vi "BC Wrapper.vi"(0 "File To Program":path, 7 "BootCommander Folder":path, 11 "Error In":errorcluster) -> (4 "StdOut":string, 6 "Std Error":string, 15 "error out":errorcluster)   [LabVIEW 2021]
doc: "It's wrapper for the BootCommander.exe"
uses:
  Controls/Console Manager Functions.ctl
  <vilib>/JKI/JKI DotNet System Exec/dotnet_system_exec/dotnet_system_exec.lvclass
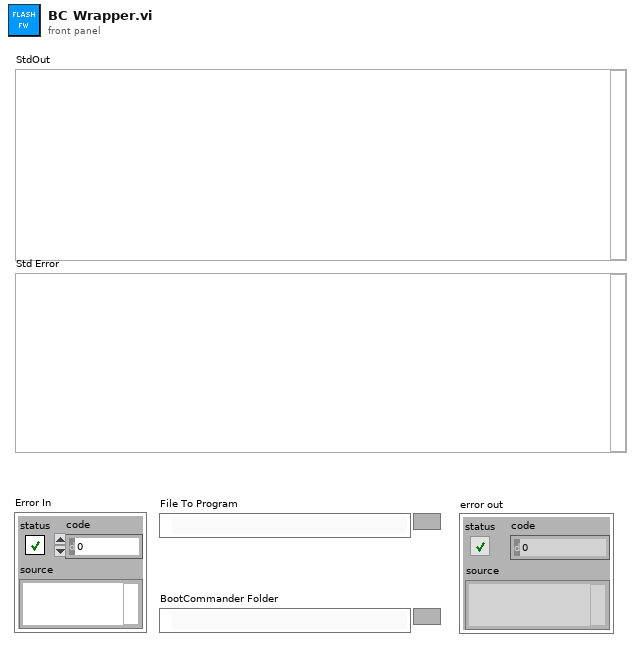
[diagram p1: front panel]
types:
  T1 = typedef "Console Manager Functions.ctl" = enum16{"Init", "Add", "Get"}
  T2 = cluster{"stdout event":refnum<user-event>, "stderr event":refnum<user-event>, "process_exit event":refnum<user-event>}
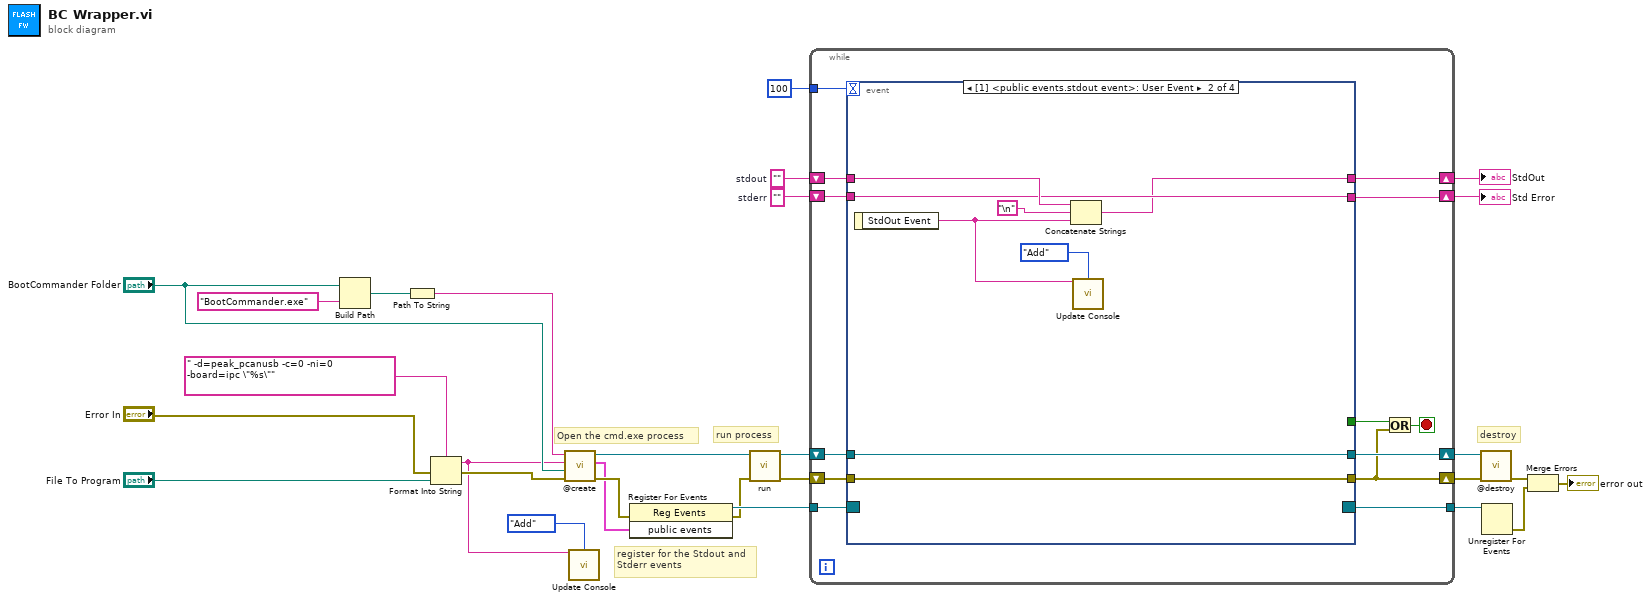
[diagram p0: block diagram]
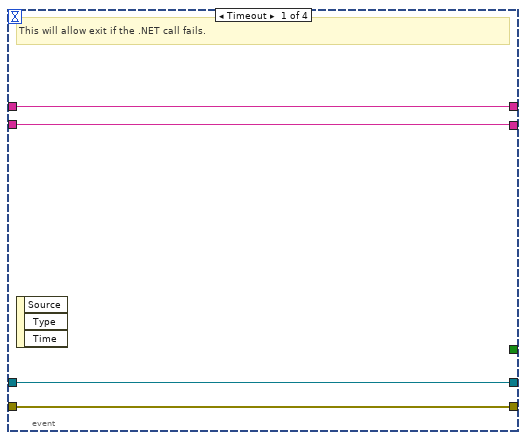
[diagram p2: hidden frame]
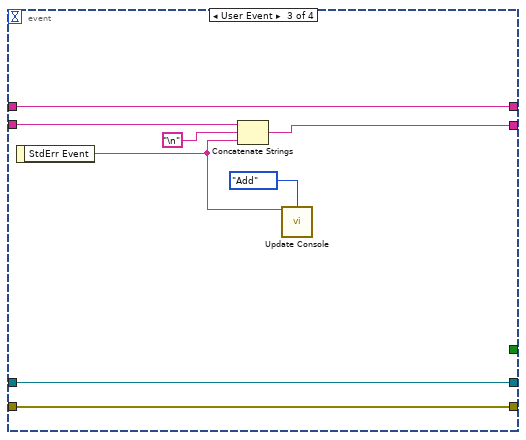
[diagram p3: hidden frame]
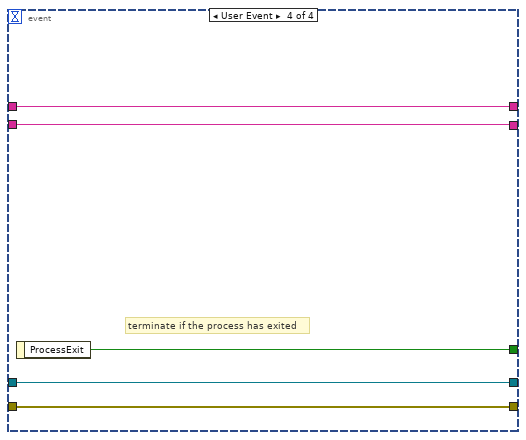
[diagram p4: hidden frame]
diagram:
  w17 = ""  # stderr
  w21 = ""  # stdout
  # "destroy"
  # "register for the Stdout and\nStderr events"
  # "run process"
  # "Open the cmd.exe process"
  n1 = Build Path(base path="BootCommander Folder", name or relative path="BootCommander.exe") -> (appended path=w10:path)
  n2 = Path To String(path=w10) -> (string=w9:string)
  n3 = Format Into String(format string=" -d=peak_pcanusb -c=0 -ni=0 -board=ipc \"%s\"" ("string"), error in="Error In", "File To Program") -> (resulting string=w1:string, error out=w7:errorcluster)  [unwired: 1 in]
  n4 = call <vilib>:"@create.vi"("error in (no error)"=w7, "working directory (c:\\)"="BootCommander Folder", "arguments (\"\")"=w1, "command line (cmd.exe)"=w9) -> ("error out"=w20:errorcluster, "public events"=w18:T2, "dotnet_system_exec out"=w27:refnum<class "dotnet_system_exec.lvclass">)  [unwired: 5 in]
  n5 = call "Update Console.vi"("New Line"=w1, "Function"=Console_Manager_Functions."Add") -> ()  [unwired: 12 in, 2 out]
  n6 = register-events(error in=w20, w18) -> (reference out=w26:refnum<event-registration>, error out=w19:errorcluster)  [unwired: 1 in]
  n7 = call <vilib>:"run.vi"("error in (no error)"=w19, "dotnet_system_exec in"=w27) -> ("error out"=w15:errorcluster, "dotnet_system_exec out"=w16:refnum<class "dotnet_system_exec.lvclass">)  [unwired: 8 in]
  n8 = while {
    shift-right: [w41] -> w28
    shift-left: w16 -> [w40]
    shift-right: [w30] -> w24
    shift-left: w15 -> [w39]
    tunnel: w26 -> [w38]
    tunnel: [w37] -> w25
    shift-right: [w35] -> w4
    shift-left: w21 -> [w36]
    shift-right: [w33] -> w3
    shift-left: w17 -> [w34]
    tunnel: 100 -> [w29]
    stop <- w32 stop-if-true
    n9 = event shown="[1] <public events.stdout event>: User Event" {
      selector: w38 -> [_ _ _ _]
      dyn-events: [_ _ _ _] -> w37
      timeout: w29 -> [_ _ _ _]
      tunnel: [w45 w53 w61 w63] -> w41
      tunnel: w40 -> [w45 w53 w61 w63]
      tunnel: w39 -> [w44 w49 w60 w62]
      tunnel: [w44 w49 w60 w62] -> w30
      tunnel: w36 -> [w43 w51 w57 w64]
      tunnel: [w43 w48 w57 w64] -> w35
      tunnel: [_ _ _ w66] -> w31
      tunnel: w34 -> [w42 w50 w58 w65]
      tunnel: [w42 w50 w56 w65] -> w33
      event Timeout {
        # "This will allow exit if the .NET call fails."
        n10 = event-data() -> ()  [unwired: 1 in, 3 out]
      }
      event User Event {
        n11 = event-data() -> ("StdOut Event"=w46:string)  [unwired: 1 in]
        n12 = Concatenate Strings(w51, "\n", w46) -> (w48:string)
        n13 = call "Update Console.vi"("New Line"=w46, "Function"=Console_Manager_Functions."Add") -> ()  [unwired: 12 in, 2 out]
      }
      event User Event {
        n14 = event-data() -> ("StdErr Event"=w54:string)  [unwired: 1 in]
        n15 = Concatenate Strings(w58, "\n", w54) -> (w56:string)
        n16 = call "Update Console.vi"("New Line"=w54, "Function"=Console_Manager_Functions."Add") -> ()  [unwired: 12 in, 2 out]
      }
      event User Event {
        # "terminate if the process has exited"
        n17 = event-data() -> ("ProcessExit"=w66:bool)  [unwired: 1 in]
      }
    }
    n18 = Or(x=w31, y=w30) -> (x .or. y?=w32:bool)
  }
  "StdOut" <- w4
  "Std Error" <- w3
  n19 = call-dynamic "@destroy.vi"("error in (no error)"=w24, "dotnet_system_exec in"=w28) -> ("error out"=w23:errorcluster)  [unwired: 8 in, 1 out]
  n20 = Unregister For Events(event registration refnum=w25) -> (error out=w22:errorcluster)  [unwired: 1 in]
  n21 = Merge Errors(w23, w22) -> (→"error out":errorcluster)
